vi "TransmitStringNoSemaphore.vi"(8 "error in (no error)":errorcluster, 10 "string to transmit":string, 11 "queue cluster":T1) -> (0 "error out":errorcluster, 3 "queue cluster out":T1)   [LabVIEW 2014]
uses:
  typedefs/QueueCluster.ctl
  typedefs/clientStatus.ctl
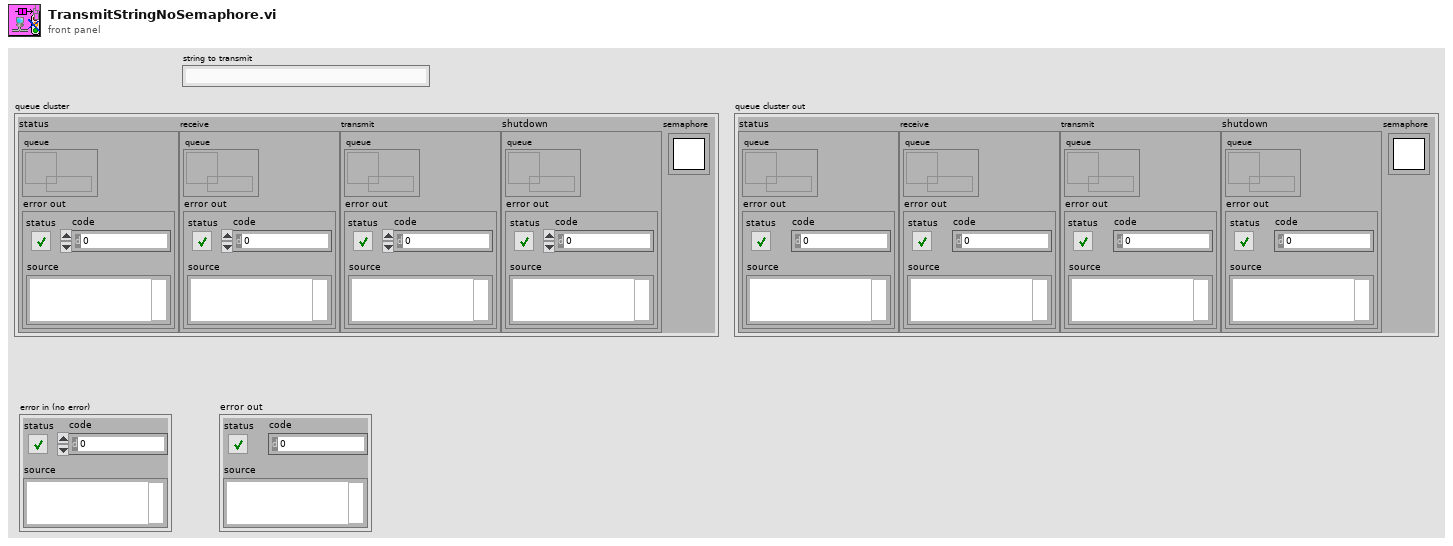
[diagram p1: front panel]
types:
  T1 = typedef "QueueCluster.ctl" = cluster{"status":cluster{"queue":refnum<queue>, "error out":errorcluster}, "receive":cluster{"queue":refnum<queue>, "error out":errorcluster}, "transmit":cluster{"queue":refnum<queue>, "error out":errorcluster}, "shutdown":cluster{"queue":refnum<queue>, "error out":errorcluster}, "semaphore":T2}
  T2 = typedef "Semaphore RefNum" = refnum<k1>
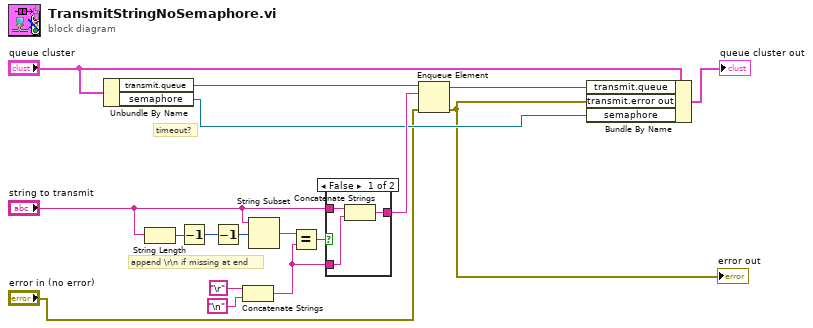
[diagram p0: block diagram]
diagram:
  # "timeout?"
  # "append \\r\\n if missing at end"
  n1 = Unbundle By Name("queue cluster") -> ("transmit.queue"=w17:refnum<queue>, "semaphore"=w3:T2)
  n2 = String Length(string="string to transmit") -> (length=w13:i32)
  n3 = Decrement(x=w13) -> (x-1=w12:i32)
  n4 = Decrement(x=w12) -> (x-1=w6:i32)
  n5 = Concatenate Strings("\r", "\n") -> (w5:string)
  n6 = String Subset(string="string to transmit", offset (0)=w6) -> (substring=w11:string)  [unwired: 1 in]
  n7 = Equal?(x=w11, y=w5) -> (x = y?=w10:bool)
  n8 = case shown="False" w10 {
    tunnel: "string to transmit" -> [w19 w21]
    tunnel: [w20 w21] -> w8
    tunnel: w5 -> [w18 _]
    frame False {
      n9 = Concatenate Strings(w19, w18) -> (w20:string)
    }
    frame True {
    }
  }
  n10 = Enqueue Element(queue=w17, element=w8, error in (no error)="error in (no error)") -> (queue out=w14:refnum<queue>, error out=w1:errorcluster)  [unwired: 1 in, 1 out]
  "error out" <- w1
  n11 = Bundle By Name(cluster="queue cluster", "transmit.queue"=w14, "transmit.error out"=w1, "semaphore"=w3) -> (→"queue cluster out":T1)
